vi "Gettimeout_raw.vi"(8 "error in (no error)":errorcluster, 11 "OneOfTemplate in":refnum<class "nixnet_grpc_WriteSignalXYRequest_timeout_enum.lvclass">) -> (0 "error out":errorcluster, 2 "Get_Val":dbl format="%.2f", 3 "OneOfTemplate out":refnum<class "nixnet_grpc_WriteSignalXYRequest_timeout_enum.lvclass">)   [LabVIEW 2019, in "xnet-grpc_client.lvlib" / "nixnet_grpc_WriteSignalXYRequest_timeout_enum.lvclass"]
uses:
  nixnet_grpc_WriteSignalXYRequest_timeout_enum.lvclass
  nixnet_grpc_WriteSignalXYRequest_timeout_enum.lvclass/nixnet_grpc_WriteSignalXYRequest_timeout_enum.ctl
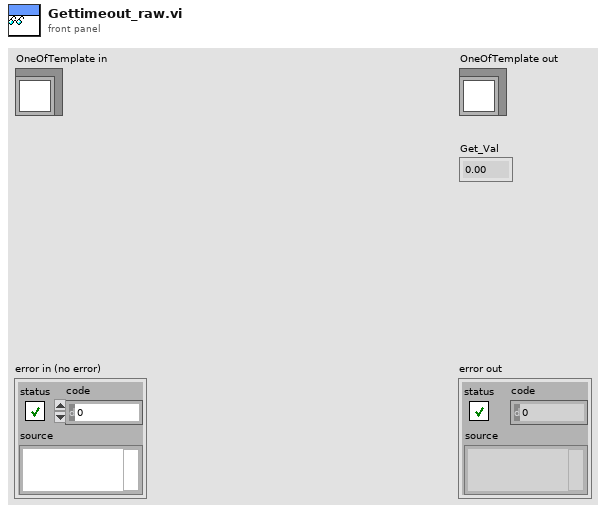
[diagram p1: front panel]
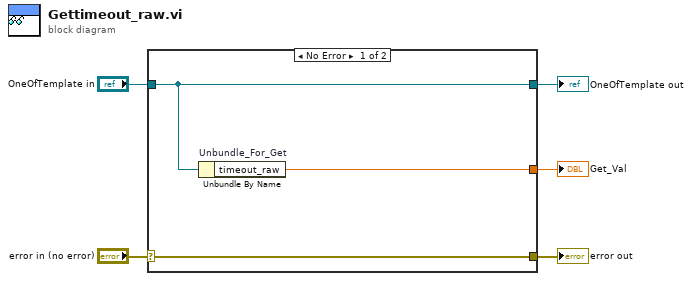
[diagram p0: block diagram]
diagram:
  n1 = case shown="No Error" "error in (no error)" {
    selector: "error in (no error)" -> [w8 w9]
    tunnel: [w8 w9] -> w4
    tunnel: [w7 w10] -> w2
    tunnel: "OneOfTemplate in" -> [w7 w10]
    tunnel: [w6 _] -> w1
    frame No Error {
      n2 = Unbundle By Name "Unbundle_For_Get"(w7) -> ("timeout_raw"=w6:dbl)
    }
    frame Error {
    }
  }
  "error out" <- w4
  "OneOfTemplate out" <- w2
  "Get_Val" <- w1
